vi "Material-Line 2-CurandPlot.vi"(0 "Material-RunTest in":refnum<class "Material-RunTest.lvclass">, 5 "error in (no error)":errorcluster) -> (14 "Material-RunTest out":refnum<class "Material-RunTest.lvclass">, 19 "error out":errorcluster)   [LabVIEW 2013, in "Material-RunTest.lvclass"]
uses:
  Material-RunTest.lvclass
  Material-RunTest.lvclass/Material-RunTest.ctl
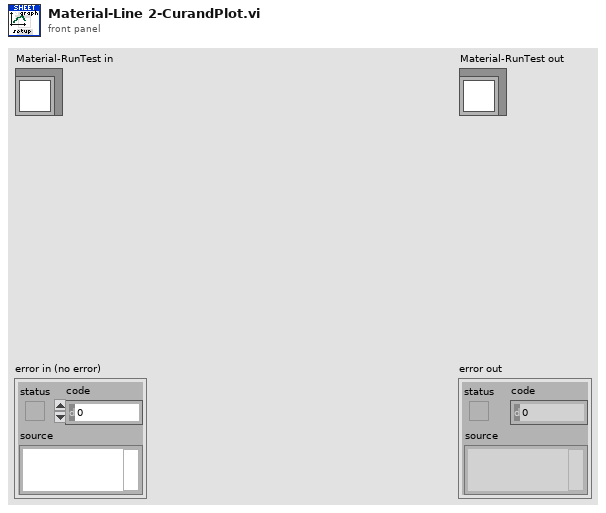
[diagram p1: front panel]
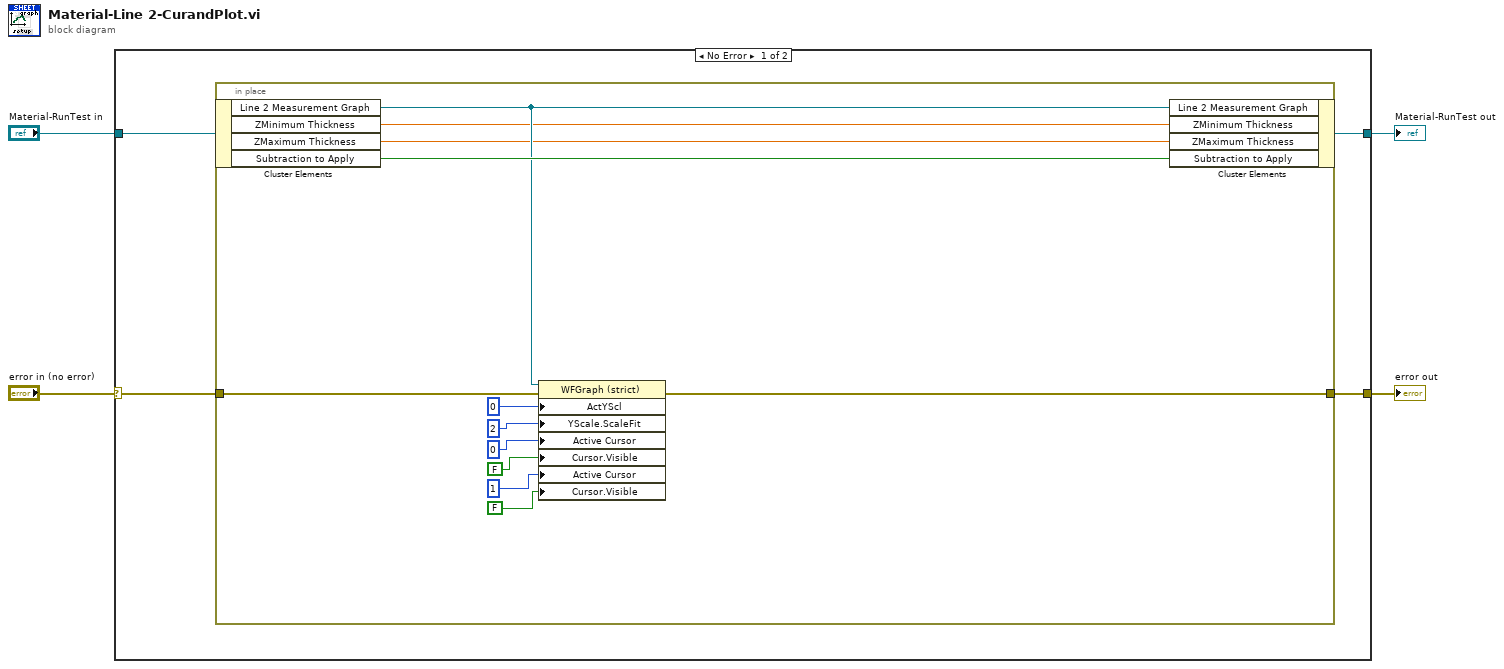
[diagram p0: block diagram]
diagram:
  n1 = case shown="No Error" "error in (no error)" {
    selector: "error in (no error)" -> [w6 w22]
    tunnel: [w5 w22] -> w3
    tunnel: [w7 w21] -> w1
    tunnel: "Material-RunTest in" -> [w8 w21]
    frame No Error {
      n2 = in-place {
        in-place-border: w6 -> [w14]
        in-place-border: [w10] -> w5
        n3 = in-place-cluster #1(w8) -> ("Line 2 Measurement Graph"=w13:refnum<vi>, "ZMinimum Thickness"=w12:dbl, "ZMaximum Thickness"=w11:dbl, "Subtraction to Apply"=w20:bool)
        n4 = property on="Property Node" class="WFGraph (strict)"(reference=w13, error in=w14, "ActYScl"=0 ("Active Y Scale"), "YScale.ScaleFit"=u8 2 ("Y Scale.Scale Fit"), "Active Cursor"=u32 0, "Cursor.Visible"=FALSE, "Active Cursor"=u32 1, "Cursor.Visible"=FALSE) -> (error out=w10:errorcluster)  [unwired: 1 out]
        n5 = in-place-cluster #1("Line 2 Measurement Graph"=w13, "ZMinimum Thickness"=w12, "ZMaximum Thickness"=w11, "Subtraction to Apply"=w20) -> (w7:refnum<class "Material-RunTest.lvclass">)
      }
    }
    frame Error {
    }
  }
  "error out" <- w3
  "Material-RunTest out" <- w1
